vi "TREE_example.vi"() -> ()   [LabVIEW 2011]
panel:
  in  "Multicolumn Listbox":i32(listbox)
  out "Active Cell":string
  in  "stop":bool
  in  "Tree":string(tree)
  in  "Start path":path
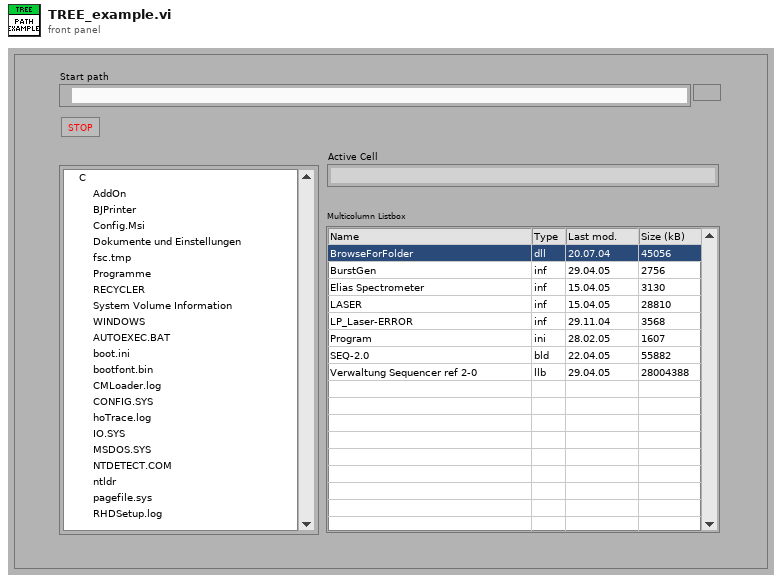
[diagram p1: front panel]
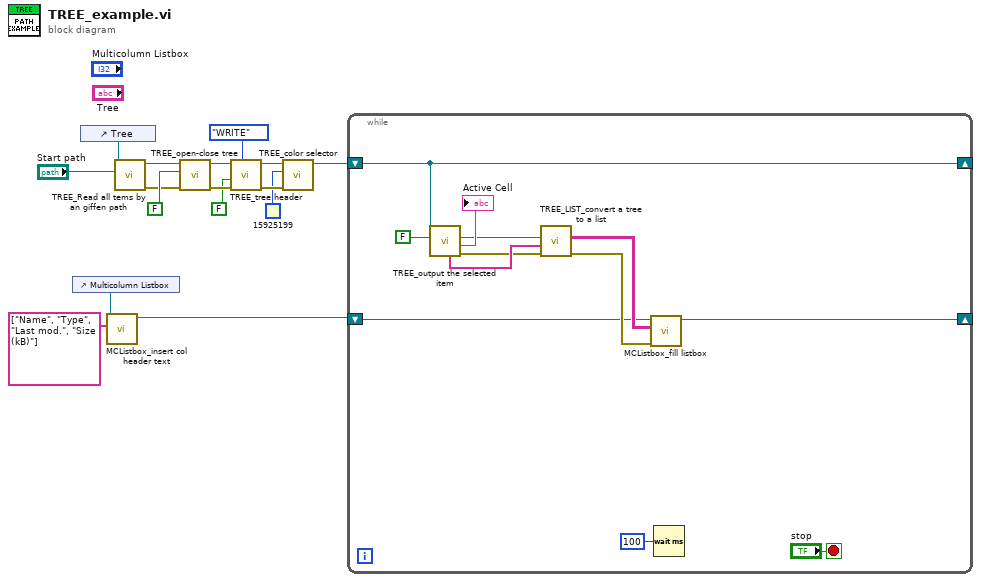
[diagram p0: block diagram]
diagram:
  n1 = control-ref of="Multicolumn Listbox"() -> (w4:refnum<vi>)
  n2 = control-ref of="Tree"() -> (w16:refnum<vi>)
  n3 = call <userlib>:"MCListbox_insert col header text.vi"("Column Header Strings"=string[] ["Name", "Type", "Last mod.", "Size (kB)"], "MCListbox in"=w4) -> ("MCListbox"=w3:refnum<vi>)  [unwired: 8 in, 1 out]
  n4 = call <userlib>:"TREE_Read all tems by an giffen path.vi"("path to start the search"="Start path", "Tree In"=w16) -> ("error out"=w13:errorcluster, "Tree Out"=w15:refnum<vi>)  [unwired: 7 in, 1 out]
  n5 = call <userlib>:"TREE_open-close tree.vi"("error in"=w13, "Open/Close tree (F=CLOSE)"=FALSE, "Tree In"=w15) -> ("error out"=w11:errorcluster, "Tree Out"=w12:refnum<vi>)  [unwired: 7 in]
  n6 = call <userlib>:"TREE_tree header.vi"("Direction"=enum16{"READ", "WRITE"}."WRITE", "error in"=w11, "Column Headers Visible (F)"=FALSE ("Column Headers Visible (T)"), "Tree In"=w12) -> ("error out"=w7:errorcluster, "Tree Out"=w8:refnum<vi>)  [unwired: 5 in, 1 out]
  n7 = call <userlib>:"TREE_color selector.vi"("error in"=w7, "Selector color"=u32 15925199, "Tree In"=w8) -> ("Tree Out"=w1:refnum<vi>)  [unwired: 7 in, 1 out]
  n8 = while {
    shift-right: [w17] -> _
    shift-left: w1 -> [w17]
    shift-right: [w18] -> _
    shift-left: w3 -> [w19]
    stop <- "stop" stop-if-true
    n9 = call <userlib>:"TREE_output the selected item.vi"("only if double click (F)"=FALSE, "Tree In"=w17) -> ("error out"=w22:errorcluster, "selected item"=→"Active Cell":string, "selectrd item (path)"=w24:path, "directory file names"=w23:string[])  [unwired: 5 in, 1 out]
    n10 = call <userlib>:"TREE_LIST_convert a tree to a list.vi"("error in (no error)"=w22, "directory file names"=w23, "selectrd item (path)"=w24) -> ("error out"=w21:errorcluster, "File info out"=w20:string[][])  [unwired: 7 in]
    n11 = call <userlib>:"MCListbox_fill listbox.vi"("error in (no error)"=w21, "Array of Strings"=w20, "MCListbox in"=w19) -> ("MCListbox"=w18:refnum<vi>)  [unwired: 7 in, 1 out]
    n12 = Wait (ms)(milliseconds to wait=u32 100) -> ()  [unwired: 1 out]
  }
